vi "ModuleManager Page.vi"(8 "?":errorcluster) -> ()   [LabVIEW 2023, in "Vires VTD System Explorer.lvlib"]
uses:
  Vires VTD System Explorer.lvlib
  <vilib>/NI VeriStand/Custom Device API/Custom Device Item Ref.ctl
  Shared/Sensor Name.ctl
  Shared/Protocol.ctl
  Shared/Timedloop Settings.ctl
  Shared/SensorInfo.ctl
  MM/MM Data.ctl
  MM/MM Objects.ctl
  MM/MM Object.ctl
  <vilib>/Utility/error.llb/Trim Whitespace One-Sided.vi
  <vilib>/NI VeriStand/Custom Device API/Custom Device API.lvlib
  Shared/Vires VTD Shared.lvlib
  MM/MM.lvlib
panel:
  in  "Tab Control":enum32{"Sensor", "Timedloop Settings"}(tab)
  in  "PlayerID":u8=1
  in  "Add Sensor":bool
  in  "# Culled Objects":i32=1
  in  "Network port":i32=48185
  in  "Protocol":T1
  in  "Sensor Name":T2
  in  "Timed Loop Settings for ModuleManager Loop":T3={"Period(ms)"=2, "Priority"=100, "Processor"=-2}
  in  "Header":cluster{"Section Name":string}={"Section Name"="Custom Device Item Settings"}
  in  "Description":string
  in  "Name":string
  in  "Node Ptr":T4 format="%.0x"
  out "error out":errorcluster
  in  "SHDocVw.IWebBrowser2":refnum<k7>(container)
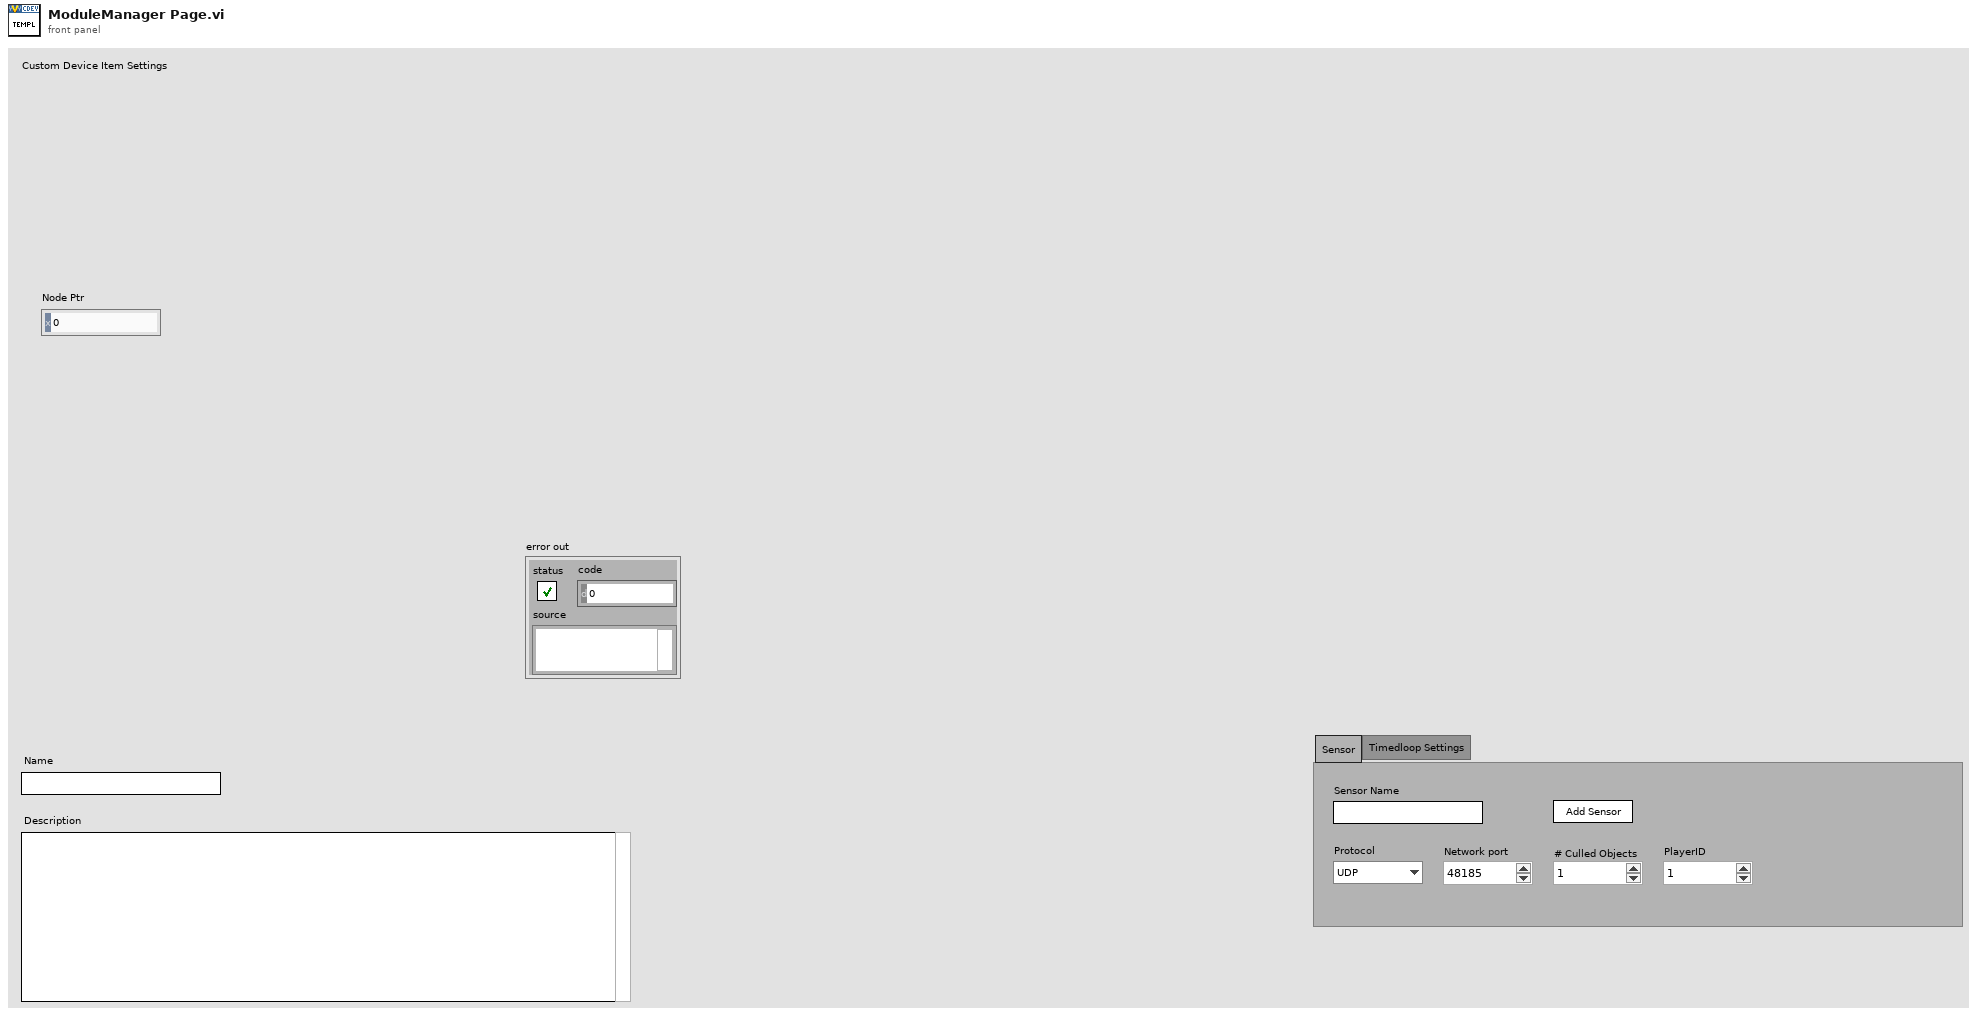
[diagram p1: front panel]
types:
  T1 = typedef "Vires VTD Shared.lvlib/Protocol.ctl" = enum16{"UDP", "TCP"}
  T2 = typedef "Vires VTD Shared.lvlib/Sensor Name.ctl" = string
  T3 = typedef "Vires VTD Shared.lvlib/Timedloop Settings.ctl" = cluster{"Period(ms)":i64, "Priority":i32, "Processor":i32}
  T4 = typedef "Custom Device API.lvlib/Custom Device Item Ref.ctl" = u64
  T5 = typedef "Custom Device API.lvlib/Custom Device Item Info.ctl" = cluster{"Name":string, "Is Channel":bool, "GUID":string, "Is Waveform":bool}
  T6 = typedef "Vires VTD Shared.lvlib/SensorInfo.ctl" = cluster{"Sensor Name":T2, "Protocol":T1, "Network port":i32, "# Culled Objects":i32, "PlayerID":u8, "MM Data":T7}
  T7 = typedef "Vires VTD Shared.lvlib/MM Data.ctl" = T8[]
  T8 = typedef "MM.lvlib/MM Objects.ctl" = cluster{"pkID":i32, "MM Objects":T9[]}
  T9 = typedef "MM.lvlib/MM Object.ctl" = cluster{"Object":i32, "Signals":string[]}
  T10 = typedef "Custom Device API.lvlib/Custom Device Commands.ctl" = enum16{"Default", "Item renamed", "Shutdown", "Dynamic button pressed"}
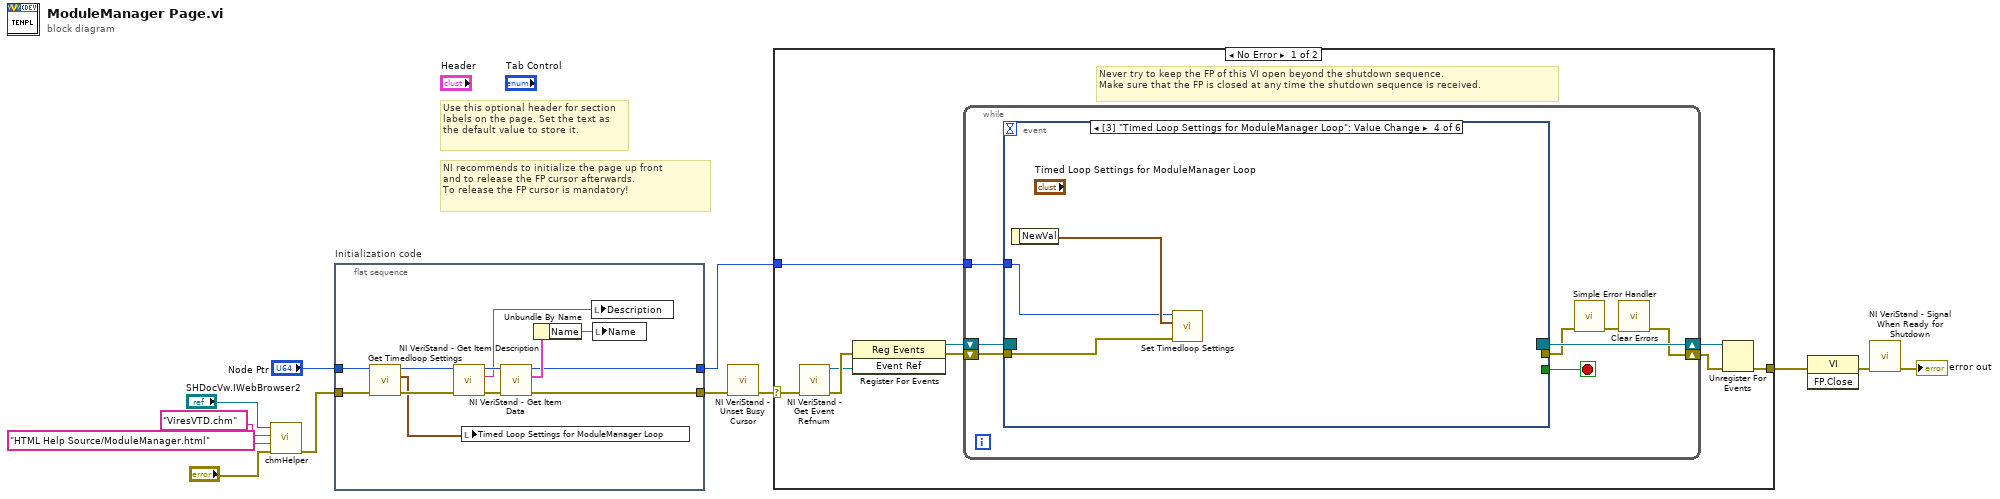
[diagram p0: block diagram]
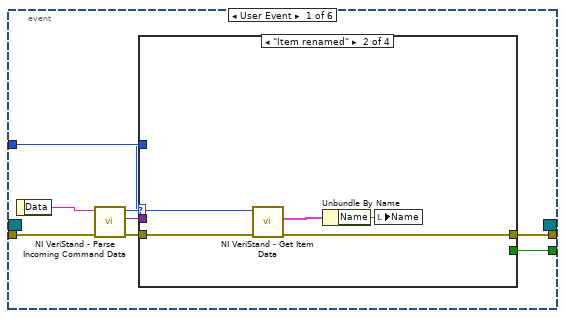
[diagram p2: hidden frame]
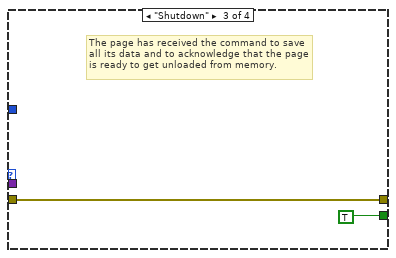
[diagram p4: hidden frame]
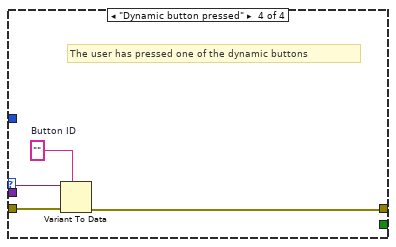
[diagram p5: hidden frame]
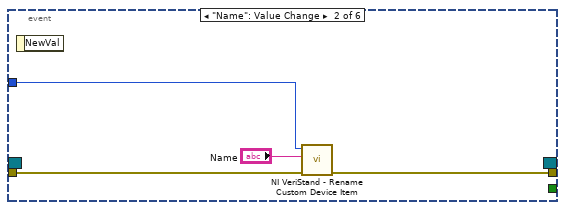
[diagram p6: hidden frame]
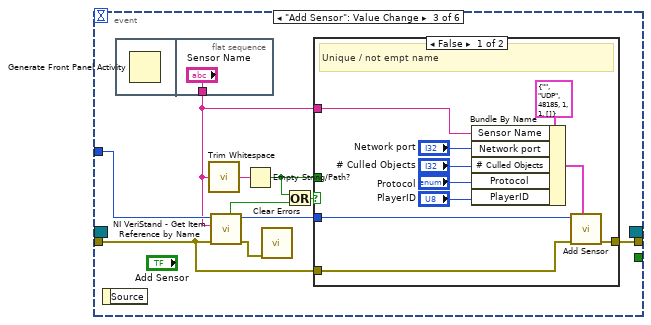
[diagram p7: hidden frame]
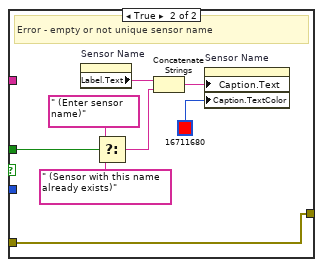
[diagram p8: hidden frame]
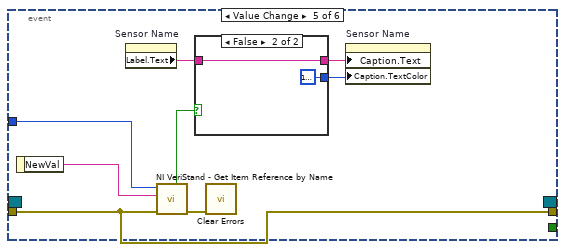
[diagram p9: hidden frame]
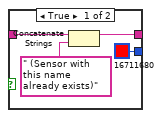
[diagram p10: hidden frame]
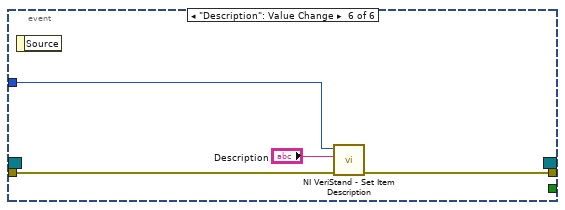
[diagram p11: hidden frame]
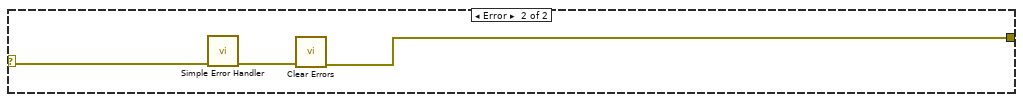
[diagram p12: hidden frame]
diagram:
  # "Use this optional header for section labels on the page. Set the text as the default value to store it."
  # "NI recommends to initialize the page up front\nand to release the FP cursor afterwards.\nTo release the FP cursor is mandatory!"
  n1 = call "chmHelper.vi"("error in (no error)"="?", "HTML File"="HTML Help Source/ModuleManager.html", "Main CHM File"="ViresVTD.chm" ("HTML File"), "Automation Refnum in"="SHDocVw.IWebBrowser2") -> ("error out"=w2:errorcluster)  [unwired: 7 in]
  n2 = flat-sequence "Initialization code" {
    tunnel: w2 -> [w17]
    tunnel: "Node Ptr" -> [w15]
    tunnel: [w20] -> w4
    tunnel: [w21] -> w1
    frame #0 {
      n3 = call "Get Timedloop Settings.vi"("error in"=w17, "Item Ref in"=w15) -> ("error out"=w16:errorcluster, "Timed Loop Settings"=w13:T3, "Item Ref out"=w14:T4)  [unwired: 7 in]
      n4 = call <vilib>:"NI VeriStand - Get Item Description.vi"("error in (no error)"=w16, "Item Ref in"=w14) -> ("error out"=w23:errorcluster, "Description"=w19:string, "Item Ref out"=w24:T4)  [unwired: 7 out]
      n5 = local write "Timed Loop Settings for ModuleManager Loop"(w13) -> ()
      n6 = call <vilib>:"NI VeriStand - Get Item Data.vi"("error in (no error)"=w23, "Item Ref in"=w24) -> ("error out"=w20:errorcluster, "Item Info"=w22:T5, "Item Ref out"=w21:T4)  [unwired: 7 out]
      n7 = Unbundle By Name(w22) -> ("Name"=w18:string)
      n8 = local write "Description"(w19) -> ()
      n9 = local write "Name"(w18) -> ()
    }
  }
  n10 = call <vilib>:"NI VeriStand - Unset Busy Cursor.vi"("error in (no error)"=w4) -> ("error out"=w3:errorcluster)  [unwired: 10 out]
  n11 = case shown="No Error" w3 {
    selector: w3 -> [w25 w118]
    tunnel: [w30 w116] -> w8
    tunnel: w1 -> [w26 _]
    frame No Error {
      # "Never try to keep the FP of this VI open beyond the shutdown sequence.\nMake sure that the FP is closed at any time the shutdown sequence is received."
      n12 = call <vilib>:"NI VeriStand - Get Event Refnum.vi"("error in (no error)"=w25) -> ("error out"=w33:errorcluster, "Event Ref"=w29:refnum<user-event>)  [unwired: 9 out]
      n13 = register-events(error in=w33, w29) -> (reference out=w27:refnum<event-registration>, error out=w28:errorcluster)  [unwired: 1 in]
      n14 = while {
        tunnel: w26 -> [w37]
        shift-right: [w34] -> w31
        shift-left: w28 -> [w40]
        shift-right: [w41] -> w32
        shift-left: w27 -> [w39]
        stop <- w38 stop-if-true
        n15 = event shown="[3] \"Timed Loop Settings for ModuleManager Loop\": Value Change" {
          selector: w39 -> [_ _ _ _ _ _]
          dyn-events: [_ _ _ _ _ _] -> w41
          timeout: _ -> [_ _ _ _ _ _]
          tunnel: w40 -> [w49 w65 w68 w95 w99 w114]
          tunnel: [w45 _ _ _ _ _] -> w38
          tunnel: [w44 w64 w75 _ w99 w113] -> w36
          tunnel: w37 -> [w43 w63 w74 w96 w105 w115]
          event User Event {
            n16 = event-data() -> ("Data"=w48:string)  [unwired: 1 out]
            n17 = call <vilib>:"NI VeriStand - Parse Incoming Command Data.vi"("error in (no error)"=w49, "Incoming data"=w48) -> ("error out"=w47:errorcluster, "Outgoing data"=w42:variant, "Action"=w46:T10)  [unwired: 7 out]
            n18 = case shown="\"Item renamed\"" w46 {
              tunnel: w47 -> [w50 w55 w56 w61]
              tunnel: [_ _ TRUE _] -> w45
              tunnel: [w50 w53 w56 w58] -> w44
              tunnel: w43 -> [_ w51 _ _]
              tunnel: w42 -> [_ _ _ w60]
              frame "Default", Default {
              }
              frame "Item renamed" {
                n19 = call <vilib>:"NI VeriStand - Get Item Data.vi"("error in (no error)"=w55, "Item Ref in"=w51) -> ("error out"=w53:errorcluster, "Item Info"=w54:T5)  [unwired: 8 out]
                n20 = Unbundle By Name(w54) -> ("Name"=w52:string)
                n21 = local write "Name"(w52) -> ()
              }
              frame "Shutdown" {
                # "The page has received the command to save all its data and to acknowledge that the page is ready to get unloaded from memory."
              }
              frame "Dynamic button pressed" {
                w59 = ""  # Button ID
                # "The user has pressed one of the dynamic buttons"
                n22 = Variant To Data(error in=w61, type=w59, Variant=w60) -> (error out=w58:errorcluster)  [unwired: 1 out]
              }
            }
          }
          event "Name": Value Change {
            n23 = event-data() -> ()  [unwired: 2 out]
            n24 = call <vilib>:"NI VeriStand - Rename Custom Device Item.vi"("error in (no error)"=w65, "New Name"="Name", "Item Ref in"=w63) -> ("error out"=w64:errorcluster)  [unwired: 1 in, 7 out]
          }
          event "Add Sensor": Value Change {
            n25 = event-data() -> ()  [unwired: 2 out]
            n26 = flat-sequence {
              tunnel: ["Sensor Name"] -> w66
              frame #0 {
                n27 = Generate Front Panel Activity() -> ()  [unwired: 1 in]
              }
              frame #1 {
              }
            }
            n28 = call <vilib>:"Trim Whitespace.vi"("string"=w66) -> ("trimmed string"=w71:string)  [unwired: 1 in]
            n29 = call <vilib>:"NI VeriStand - Get Item Reference by Name.vi"("error in (no error)"=w68, "Item Name"=w66, "Parent Ref in"=w74) -> ("error out"=w67:errorcluster, "Parent Ref out"=w73:T4, "Found"=w72:bool)  [unwired: 5 in, 1 out]
            n30 = Empty String/Path?(string/path=w71) -> (empty?=w69:bool)
            n31 = call <vilib>:"Clear Errors.vi"("error in (no error)"=w67) -> ()  [unwired: 1 in, 6 out]
            n32 = Or(x=w69, y=w72) -> (x .or. y?=w70:bool)
            n33 = case shown="False" w70 {
              tunnel: [w86 w87] -> w75
              tunnel: w73 -> [w85 _]
              tunnel: w66 -> [w78 _]
              tunnel: w69 -> [_ w88]
              tunnel: w68 -> [w77 w87]
              frame False {
                # "Unique / not empt name"
                n34 = Bundle By Name(cluster=T6 {"Sensor Name"="", "Protocol"=enum."UDP", "Network port"=48185, "# Culled Objects"=1, "PlayerID"=1, "MM Data"=[]} ("SensorInfo"), "Sensor Name"=w78, "Network port"="Network port", "# Culled Objects"="# Culled Objects", "Protocol"="Protocol", "PlayerID"="PlayerID") -> (w79:T6)
                n35 = call "Add Sensor.vi"("SensorInfo"=w79, "error in (no error)"=w77, "Item Ref in"=w85) -> ("error out (no error)"=w86:errorcluster)  [unwired: 8 in]
              }
              frame True {
                # "Error - empty or not unique sensor name"
                n36 = property on="Sensor Name" class="Str (strict)"() -> ("Label.Text"=w93:string)  [unwired: 2 in, 2 out]
                n37 = Select(t=" (Enter sensor name)" ("string"), s=w88, f=" (Sensor with this name already exists)" ("string")) -> (s? t:f=w91:string)
                n38 = Concatenate Strings(w93, w91) -> (w94:string)
                n39 = property on="Sensor Name" class="Str (strict)"("Caption.Text"=w94, "Caption.TextColor"=u32 16711680) -> ()  [unwired: 2 in, 2 out]
              }
            }
          }
          event Value Change {
            n40 = event-data() -> ("NewVal"=w97:T3)  [unwired: 1 out]
            n41 = call "Set Timedloop Settings.vi"("error in"=w95, "Timed Loop Settings"=w97, "Item Ref in"=w96) -> ()  [unwired: 7 in, 2 out]
          }
          event Value Change {
            n42 = event-data() -> ("NewVal"=w104:T2)  [unwired: 1 out]
            n43 = property on="Sensor Name" class="Str (strict)"() -> ("Label.Text"=w101:string)  [unwired: 2 in, 2 out]
            n44 = call <vilib>:"NI VeriStand - Get Item Reference by Name.vi"("error in (no error)"=w99, "Item Name"=w104, "Parent Ref in"=w105) -> ("error out"=w98:errorcluster, "Found"=w103:bool)  [unwired: 5 in, 2 out]
            n45 = case shown="False" w103 {
              tunnel: [u32 16711680 u32 16777222] -> w100
              tunnel: [w107 w110] -> w102
              tunnel: w101 -> [w108 w110]
              frame True {
                n46 = Concatenate Strings(w108, " (Sensor with this name already exists)" ("string")) -> (w107:string)
              }
              frame False {
              }
            }
            n47 = call <vilib>:"Clear Errors.vi"("error in (no error)"=w98) -> ()  [unwired: 1 in, 6 out]
            n48 = property on="Sensor Name" class="Str (strict)"("Caption.Text"=w102, "Caption.TextColor"=w100) -> ()  [unwired: 2 in, 2 out]
          }
          event "Description": Value Change {
            n49 = event-data() -> ()  [unwired: 2 out]
            n50 = call <vilib>:"NI VeriStand - Set Item Description.vi"("error in (no error)"=w114, "Description"="Description", "Item Ref in"=w115) -> ("error out"=w113:errorcluster)  [unwired: 8 out]
          }
        }
        n51 = call <vilib>:"Simple Error Handler.vi"("error in (no error)"=w36) -> ("error out"=w35:errorcluster)  [unwired: 1 in, 7 out]
        n52 = call <vilib>:"Clear Errors.vi"("error in (no error)"=w35) -> ("error out"=w34:errorcluster)  [unwired: 1 in, 5 out]
      }
      n53 = Unregister For Events(event registration refnum=w32, error in=w31) -> (error out=w30:errorcluster)
    }
    frame Error {
      n54 = call <vilib>:"Simple Error Handler.vi"("error in (no error)"=w118) -> ("error out"=w117:errorcluster)  [unwired: 1 in, 7 out]
      n55 = call <vilib>:"Clear Errors.vi"("error in (no error)"=w117) -> ("error out"=w116:errorcluster)  [unwired: 1 in, 5 out]
    }
  }
  n56 = invoke class="VI" method="FP.Close"(error in=w8) -> (error out=w7:errorcluster)  [unwired: 2 in, 2 out]
  n57 = call <vilib>:"NI VeriStand - Signal When Ready for Shutdown.vi"("error in (no error)"=w7) -> ("error out"=→"error out":errorcluster)  [unwired: 10 out]
